vi "FindExtinctionAndSizeParameterFactors.vi"(3 "output control":T4, 4 "data":T5, 5 "X":dbl[](array[numeric])) -> (0 "error out":errorcluster, 1 "gradient":dbl[](array[numeric]), 2 "f(X)":dbl)   [LabVIEW 2013]
doc: "This template is the starting point for creating an objectivel function to be passed to the Unconstrained Optimization.vi."
uses:
  <vilib>/gmath/NumericalOptimization/objective function data.ctl
  ReadBaesDataTypeDefinition.ctl
  ParticleDistributionData.ctl
  <vilib>/gmath/NI_Gmath.lvlib
panel:
  out "Size parameter Factor":dbl
  in  "Data for RIRetrieval VI":T3={"Approximate Errors"=FALSE, "Extinction ExtinctionUncertainity Size parameter and Number ofS sizes"={"Extinction"=[], "Extinction Uncertainty"=[], "Size parameters"=[], "Number ofSizes"=0.0, "GeometricCrossSection"=[], "WaveLength"=[], "Sizes"=[], "Concentration (#/cc)"=[]}, "Minimization method"=0, "Graph Ref"={"Real Part vs wavelength"=refnum, "Imaginary Part vs wavelength"=refnum, "Normalized Residuals vs Size parameter"=refnum, "Not Corrected for Multiple charge particles"=refnum, "Simplex 2"=refnum}, "Particle Distribution Data"={"SMPS Sizes"=[], "Concentration"=[], "Double Charge Correction Flag"=FALSE}, "Calculate Errors"=FALSE, "Restrict to Positive Imaginary Part"=FALSE, "MinMaxWavelength"={0, 0, "Extinction Factor"=FALSE, "Size Parameter Factor"=FALSE, "Size Parameter Offset"=TRUE, "Extinction Factor 2"=1.0, "Diameter Factor"=1.0, "Diameter Offset"=0.0, "ExtinctionOrAbsorptionOrScattering"=0}} {"MinMaxWavelength"."ExtinctionOrAbsorptionOrScattering" scale=0.0..2.0}
  out "Extinction factor":dbl
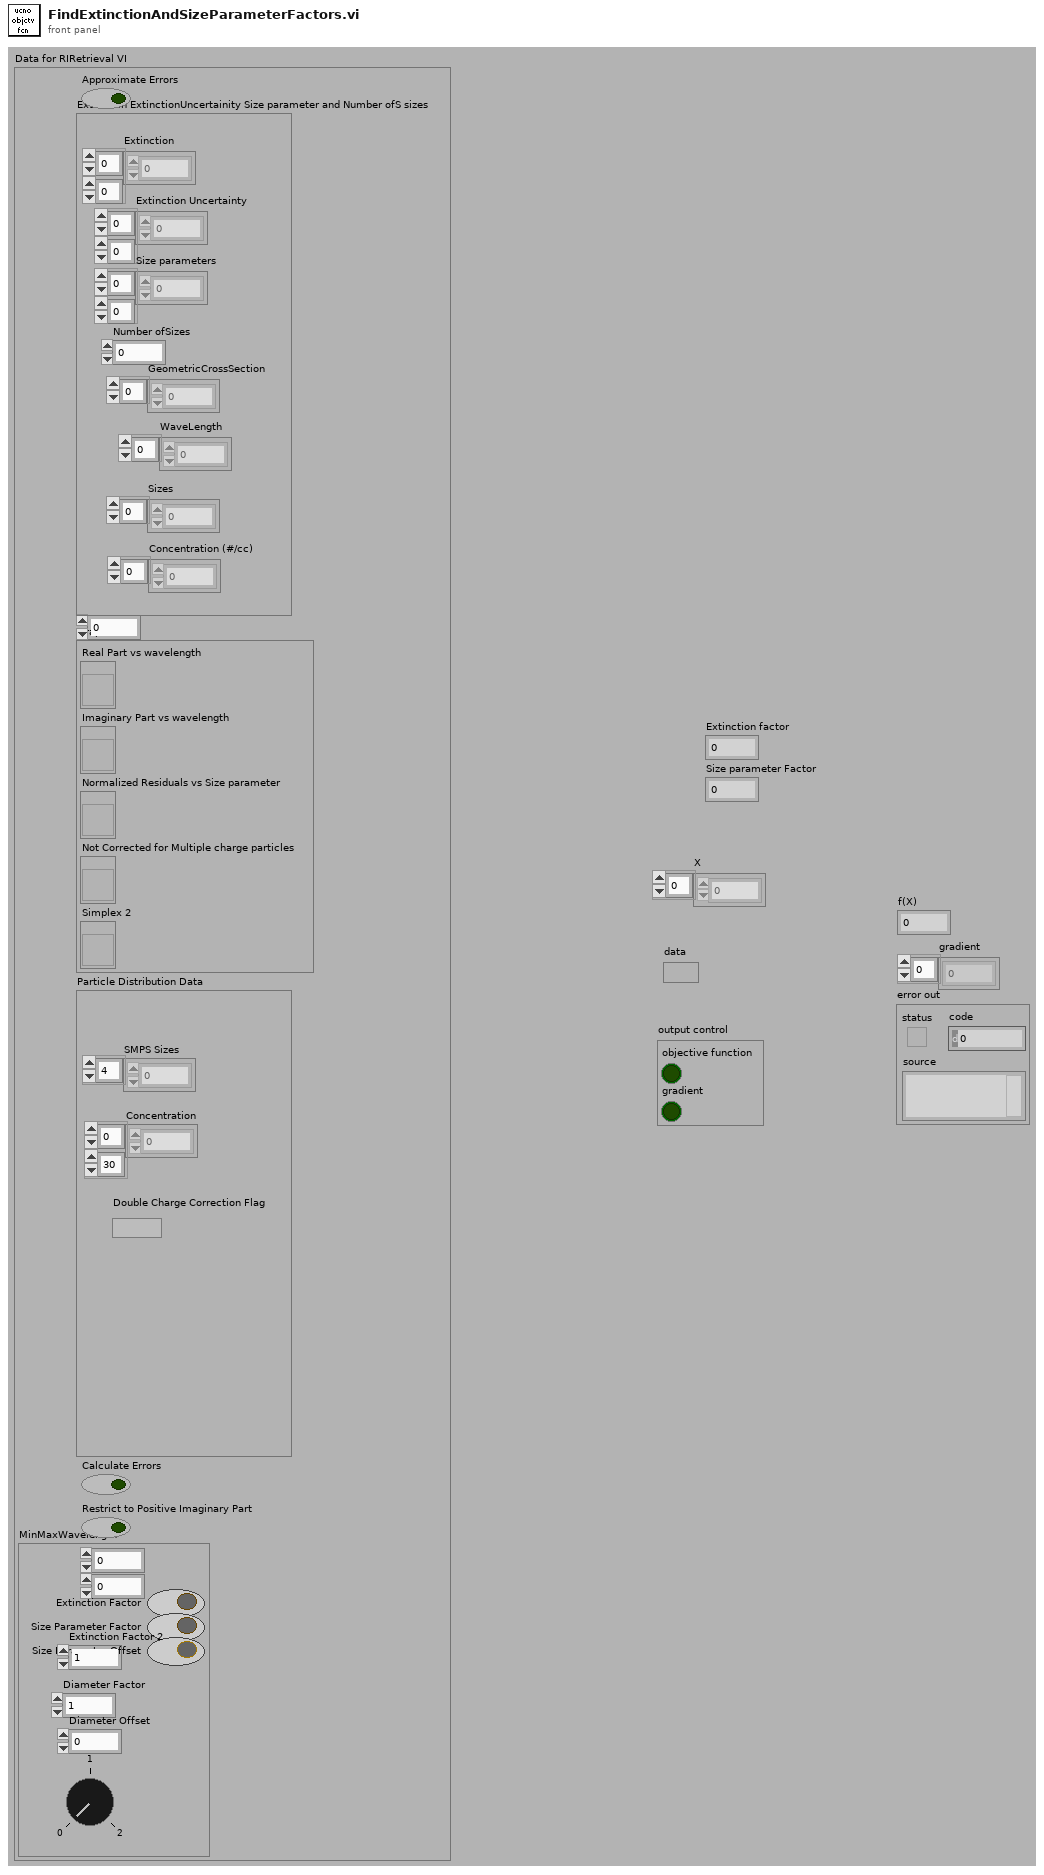
[diagram p1: front panel]
types:
  T1 = typedef "ReadBaesDataTypeDefinition.ctl" = cluster{"Extinction":dbl[][], "Extinction Uncertainty":dbl[][], "Size parameters":dbl[][], "Number ofSizes":dbl, "GeometricCrossSection":dbl[], "WaveLength":dbl[], "Sizes":dbl[], "Concentration (#/cc)":dbl[]}
  T2 = typedef "ParticleDistributionData.ctl" = cluster{"SMPS Sizes":dbl[], "Concentration":dbl[][], "Double Charge Correction Flag":bool}
  T3 = cluster{"Approximate Errors":bool, "Extinction ExtinctionUncertainity Size parameter and Number ofS sizes":T1, "Minimization method":u16, "Graph Ref":cluster{"Real Part vs wavelength":refnum<vi>, "Imaginary Part vs wavelength":refnum<vi>, "Normalized Residuals vs Size parameter":refnum<vi>, "Not Corrected for Multiple charge particles":refnum<vi>, "Simplex 2":refnum<vi>}, "Particle Distribution Data":T2, "Calculate Errors":bool, "Restrict to Positive Imaginary Part":bool, "MinMaxWavelength":cluster{i32, i32, "Extinction Factor":bool, "Size Parameter Factor":bool, "Size Parameter Offset":bool, "Extinction Factor 2":dbl, "Diameter Factor":dbl, "Diameter Offset":dbl, "ExtinctionOrAbsorptionOrScattering":i8}}
  T4 = cluster{"objective function":bool, "gradient":bool}
  T5 = typedef "NI_Gmath.lvlib/objective function data.ctl" = variant
  T6 = cluster{"Real Part vs wavelength":refnum<vi>, "Imaginary Part vs wavelength":refnum<vi>, "Normalized Residuals vs Size parameter":refnum<vi>, "Not Corrected for Multiple charge particles":refnum<vi>, "Simplex 2":refnum<vi>}
  T7 = cluster{i32, i32, "Extinction Factor":bool, "Size Parameter Factor":bool, "Size Parameter Offset":bool, "Extinction Factor 2":dbl, "Diameter Factor":dbl, "Diameter Offset":dbl, "ExtinctionOrAbsorptionOrScattering":i8}
  T8 = typedef "RIandRIMCResults.ctl" = cluster{"Real RI":dbl[], "Imaginary RI":dbl[], "Std Imaginary RI":dbl[], "Std Real RI":dbl[], "Wavelength":dbl[], "Residue":dbl[], "Extinction Factor":dbl[], "Diameter Factor":dbl[], "Diameter Offset":dbl[], "Best fit result":dbl[][], "Normalized Residuals":dbl[][]}
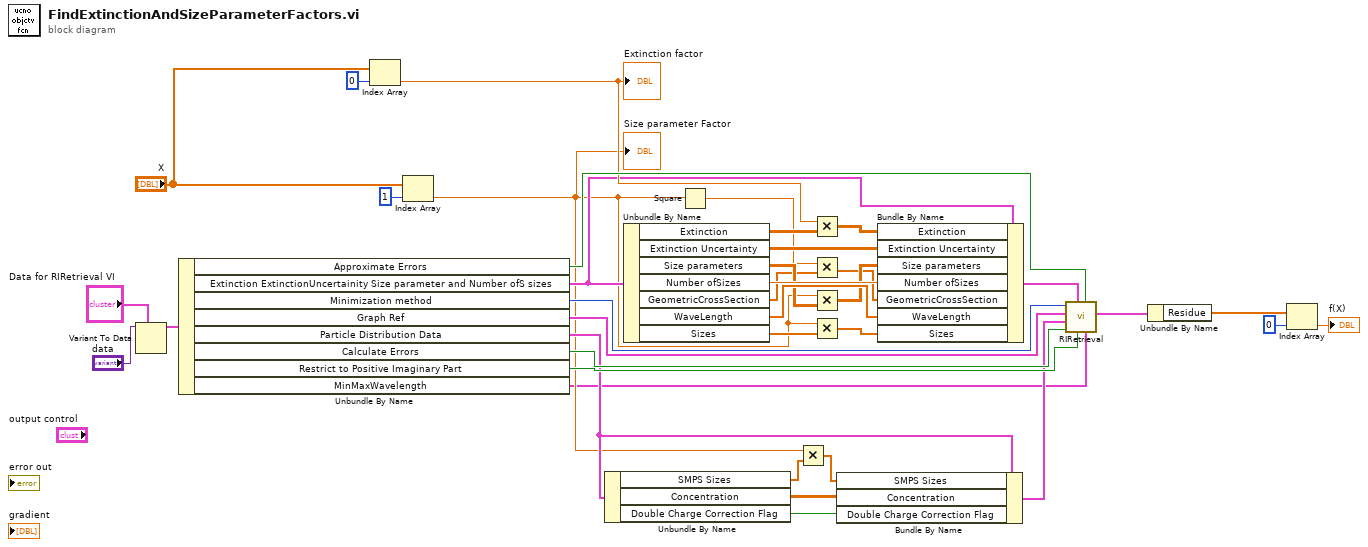
[diagram p0: block diagram]
diagram:
  n1 = Variant To Data(type="Data for RIRetrieval VI", Variant="data") -> (data=w38:T3)  [unwired: 1 in, 1 out]
  n2 = Unbundle By Name(w38) -> ("Approximate Errors"=w34:bool, "Extinction ExtinctionUncertainity Size parameter and Number ofS sizes"=w27:T1, "Minimization method"=w33:u16, "Graph Ref"=w32:T6, "Particle Distribution Data"=w8:T2, "Calculate Errors"=w31:bool, "Restrict to Positive Imaginary Part"=w30:bool, "MinMaxWavelength"=w1:T7)
  n3 = Index Array(array="X", index=0) -> (element=w29:dbl)
  "Extinction factor" <- w29
  n4 = Index Array(array="X", index=1) -> (element=w3:dbl)
  "Size parameter Factor" <- w3
  n5 = Unbundle By Name(w8) -> ("SMPS Sizes"=w5:dbl[], "Concentration"=w7:dbl[][], "Double Charge Correction Flag"=w6:bool)
  n6 = Unbundle By Name(w27) -> ("Extinction"=w28:dbl[][], "Extinction Uncertainty"=w25:dbl[][], "Size parameters"=w15:dbl[][], "Number ofSizes"=w24:dbl, "GeometricCrossSection"=w12:dbl[], "WaveLength"=w23:dbl[], "Sizes"=w10:dbl[])
  n7 = Square(x=w3) -> (x^2=w13:dbl)
  n8 = Multiply(x=w3, y=w5) -> (x*y=w4:dbl[])
  n9 = Multiply(x=w29, y=w28) -> (x*y=w26:dbl[][])
  n10 = Multiply(x=w13, y=w12) -> (x*y=w11:dbl[])
  n11 = Multiply(x=w3, y=w15) -> (x*y=w14:dbl[][])
  n12 = Multiply(x=w3, y=w10) -> (x*y=w9:dbl[])
  n13 = Bundle By Name(cluster=w8, "SMPS Sizes"=w4, "Concentration"=w7, "Double Charge Correction Flag"=w6) -> (w2:T2)
  n14 = Bundle By Name(cluster=w27, "Extinction"=w26, "Extinction Uncertainty"=w25, "Size parameters"=w14, "Number ofSizes"=w24, "GeometricCrossSection"=w11, "WaveLength"=w23, "Sizes"=w9) -> (w22:T1)
  n15 = call "RIRetrieval.vi"("General Data for RI Retrieval VI"=w1, "Approximate Errors"=w34, "Restrict to Positive Imaginary Part"=w30, "Extinction Measured Data"=w22, "Calculate Errors"=w31, "Particle Distribution Data"=w2, "Graph Refs"=w32, "Minimization method"=w33) -> ("RI results"=w21:T8)  [unwired: 3 out]
  n16 = Unbundle By Name(w21) -> ("Residue"=w20:dbl[])
  n17 = Index Array(array=w20, index=0) -> (element=→"f(X)":dbl)
